vi "Valid Resource Message.vi"(8 "error in (no error)":errorcluster, 11 "Generic Optimizer in":refnum<class "Generic Optimizer.lvclass">) -> (0 "error out":errorcluster, 2 "Valid Resource Message":T1, 3 "Generic Optimizer out":refnum<class "Generic Optimizer.lvclass">)   [LabVIEW 2020, in "RxnRover.lvlib" / "Generic Optimizer.lvclass"]
uses:
  Generic Optimizer.lvclass
  <userlib>/RxnRover/DynamicReentrant/src/Type Defs/Message.ctl
  <userlib>/RxnRover/DynamicReentrant/Dynamic Reentrant.lvlib
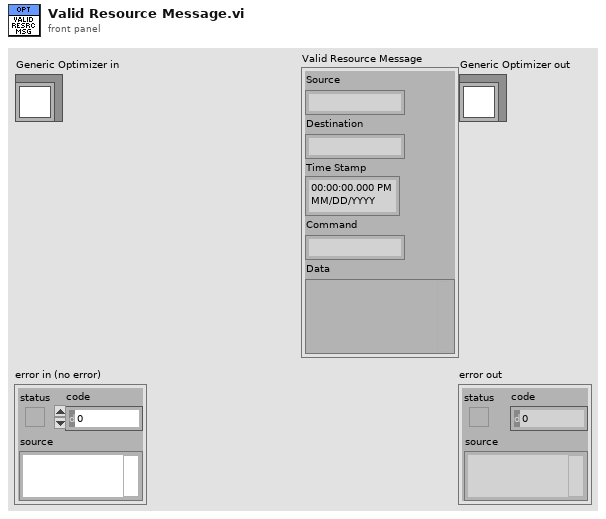
[diagram p1: front panel]
types:
  T1 = typedef "Dynamic Reentrant.lvlib/Message.ctl" = cluster{"Source":string, "Destination":string, "Time Stamp":timestamp, "Command":string, "Data":variant}
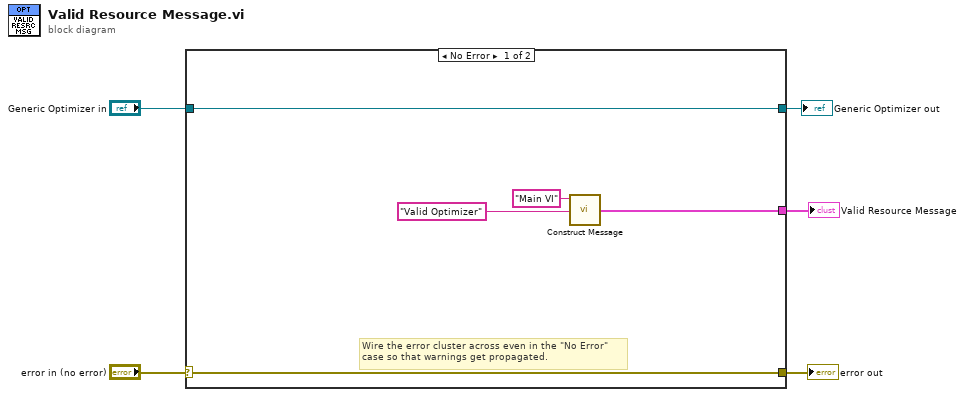
[diagram p0: block diagram]
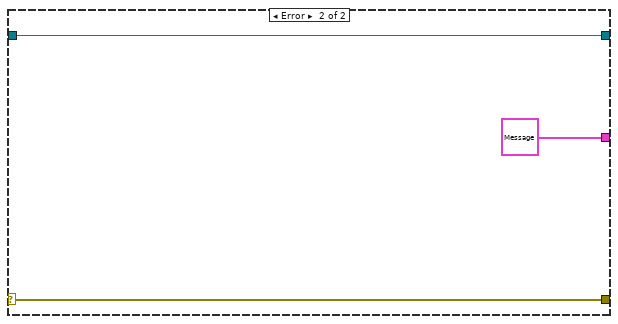
[diagram p2: hidden frame]
diagram:
  n1 = case shown="No Error" "error in (no error)" {
    selector: "error in (no error)" -> [w9 w13]
    tunnel: [w9 w13] -> w5
    tunnel: [w10 w12] -> w3
    tunnel: "Generic Optimizer in" -> [w10 w12]
    tunnel: [w6 T1 {"Source"="", "Destination"="", "Time Stamp"=timestamp(0 s since 1904-01-01), "Command"="", "Data"=variant} ("Message")] -> w4
    frame No Error {
      # "Wire the error cluster across even in the \"No Error\"\ncase so that warnings get propagated."
      n2 = call <userlib>:"Construct Message.vi"("Command"="Valid Optimizer", "Source"="Main VI") -> ("Message Cluster"=w6:T1)  [unwired: 4 in]
    }
    frame Error {
    }
  }
  "error out" <- w5
  "Generic Optimizer out" <- w3
  "Valid Resource Message" <- w4
